vi "信号光谱2_test.vi"() -> ()   [LabVIEW 2018]
uses:
  <vilib>/Analysis/NI_AALBase.lvlib
  <vilib>/Utility/file.llb/Write Delimited Spreadsheet (DBL).vi
panel:
  in  "端口":u16
  in  "地址":string
  out "configure error out":errorcluster
  out "最终存储路径":path
  in  "停止程序":bool
  in  "上升下降沿/s":dbl format="%.2p"
  in  "延时/s":dbl format="%.2p"
  in  "占空比/%":dbl=3.0 format="%.2p"
  in  "高电平/V":dbl=4.0 format="%.2p"
  in  "频率/Hz":dbl=100.0 format="%.3p"
  in  "低电平/V":dbl min=0.0 max=5.0 format="%.2p"
  in  "设置参数":bool
  out "output control error  4":errorcluster
  in  "低电平持续输出":bool
  in  "Output 1":bool
  out "output control error  5":errorcluster
  in  "脉冲作用时间/s":dbl=1.0
  in  "测量高电平/V":dbl=4.0
  out "output control error  2":errorcluster
  in  "测量次数":i32=1
  in  "开始测量":bool
  in  "上升下降沿":i32(ring)=1 items=["上升沿", "下降沿"]
  in  "channel输出口":i32(ring) items=["Channel 1", "Channel 2"]
  in  "输出信号波形":u16(ring) items=["Pulse"]
  out "output control error  3":errorcluster
  out "Output":bool
  in  "VISA 信号发生器":refnum<visa-resource-name>="USB0::0x1AB1::0x0641::DG4E192200870::INSTR"
  out "Spectrum":cluster{"Y":dbl[], "Y":dbl[]}[](graph)
  in  "计数器":dbl=720.0
  out "波长范围":dbl[](array[numeric])
  in  "选项卡控件":enum32{"IHR 550", "CCD"}(tab)
  in  "Move To\nTarget Positions":bool
  out "Current UniqueID":string="Mono4"
  in  "Mono ID":string(combo)="Mono1"
  in  "Connect":bool
  out "Initialized JY":bool=TRUE
  in  "Force\nInitialization":bool
  in  "Target Grating":string(combo)="2"
  out "Current Description":string="1" caption="Description"
  out "Grating Index":i32=1
  out "Current Grating":dbl=1200.0
  out "Units":string="nm"
  out "Current WL":dbl=897.9988
  out "Exit Mirror\nPosition":i32(ring)=2 items=["EntranceMirror", "ExitMirror", "Front", "Side"]
  out "Entrance Mirror\nPosition":i32(ring)=2 items=["EntranceMirror", "ExitMirror", "Front", "Side"]
  out "Units 2":string="mm"
  out "Front Entrance":dbl
  in  "Target WL":dbl=2670.0
  in  "Exit Mirror":u16(ring)=3 caption="Target Position Exit Mirror" items=["Front"=2, "Side"=3]
  in  "Entrance Mirror":u16(ring)=2 caption="Target Position\nEntrance Mirror" items=["Front"=2, "Side"=3]
  in  "Target\nFront Entrance":dbl=1.0
  in  "Commande tab":T1(tab)
  in  "Area Number to Display":i32
  in  "Reformat":bool
  in  "GAIN":u16(ring)=2 caption="Device Name" items=["High Light", "Best Dynamic Range", "High Sensitivity"]
  in  "ADC":u16(ring) caption="Device Name" items=["20 kHz       ", " 1 MHz       ", " 1 MHz Ultra "]
  in  "Number of Areas :":u16=1 min=1 step=1
  in  "Integration time (ms) :":i32=5000
  out "Uniques ID":u16(ring) items=["CCD1", "CCD2"]
  in  "Device Name":u16(ring) items=["Synapse CCD (Lateral)", "Synapse_IGA (Axial)"]
  in  "Signal type :":enum16{"TTL Rising Edge", "TTL Falling Edge"}(ring)=enum."TTL Falling Edge"
  in  "Trigger Type :":u16(ring) items=["On Start"=1, "Per Acquisition"=2]
  in  "trigSigTypeString":string
  in  "trigEventString":string
  in  "Enable InputTriggers :":bool
  in  "Number of Cleans":i32=1
  in  "MultiAcqShutterMode":i32(ring)=3 items=["Open For All Spectra"=1, "Open for Each Spectrum"=3]
  in  "Accumulations:":u16=10 min=1 step=1
  in  "Multi Accumulation mode:":bool
  out "Y Pixels:":i32=256
  out "DataSize":i32=1024
  out "X Pixels:":i32=1024
  out "Firmware\nVersion":string="V1.20 CCD_4000"
  out "initialized ?":bool=TRUE
  in  "Continuous":bool
  in  "CCD Busy":bool
  out "indicator":string="Ready !"
  in  "initialize":bool
  in  "ShutterOpen":bool=TRUE caption="Shutter enable"
  in  "Save Backlight":bool
  in  "Acquire":bool
  in  "Temperature":bool
  in  "Setup":bool
  in  "起始波长":dbl=2406.79
  in  "终止波长":dbl=2919.91
  out "Acq Time(ms)":u32=3401
  in  "Close":bool=TRUE
  out "JYCCDLib.IJYCCDReqd":refnum<k7>
  out "areas :":i32[][](array[numeric])=[[1], [1], [1], [1024], [256], [1], [256]]
  in  "Constante de condition\n(Voir l'aide contextuelle)":bool
  out "temp graph":dbl(graph)=-134.538067
  out "ADC Number":i32[](array[numeric])=[0, 1, 2, 3, 4]
  out "Gain Number":i32[](array[numeric])=[10, 11, 12, 13, 8, 2]
  out "trigAddress":i32
  out "Data":i32[][](graph)
  out "error out":errorcluster
  out "Gratings":dbl[](array[numeric])=[1200.0, 300.0]
  out "Backlight":i32[][](graph)
  out "data 2":i32[][](graph)
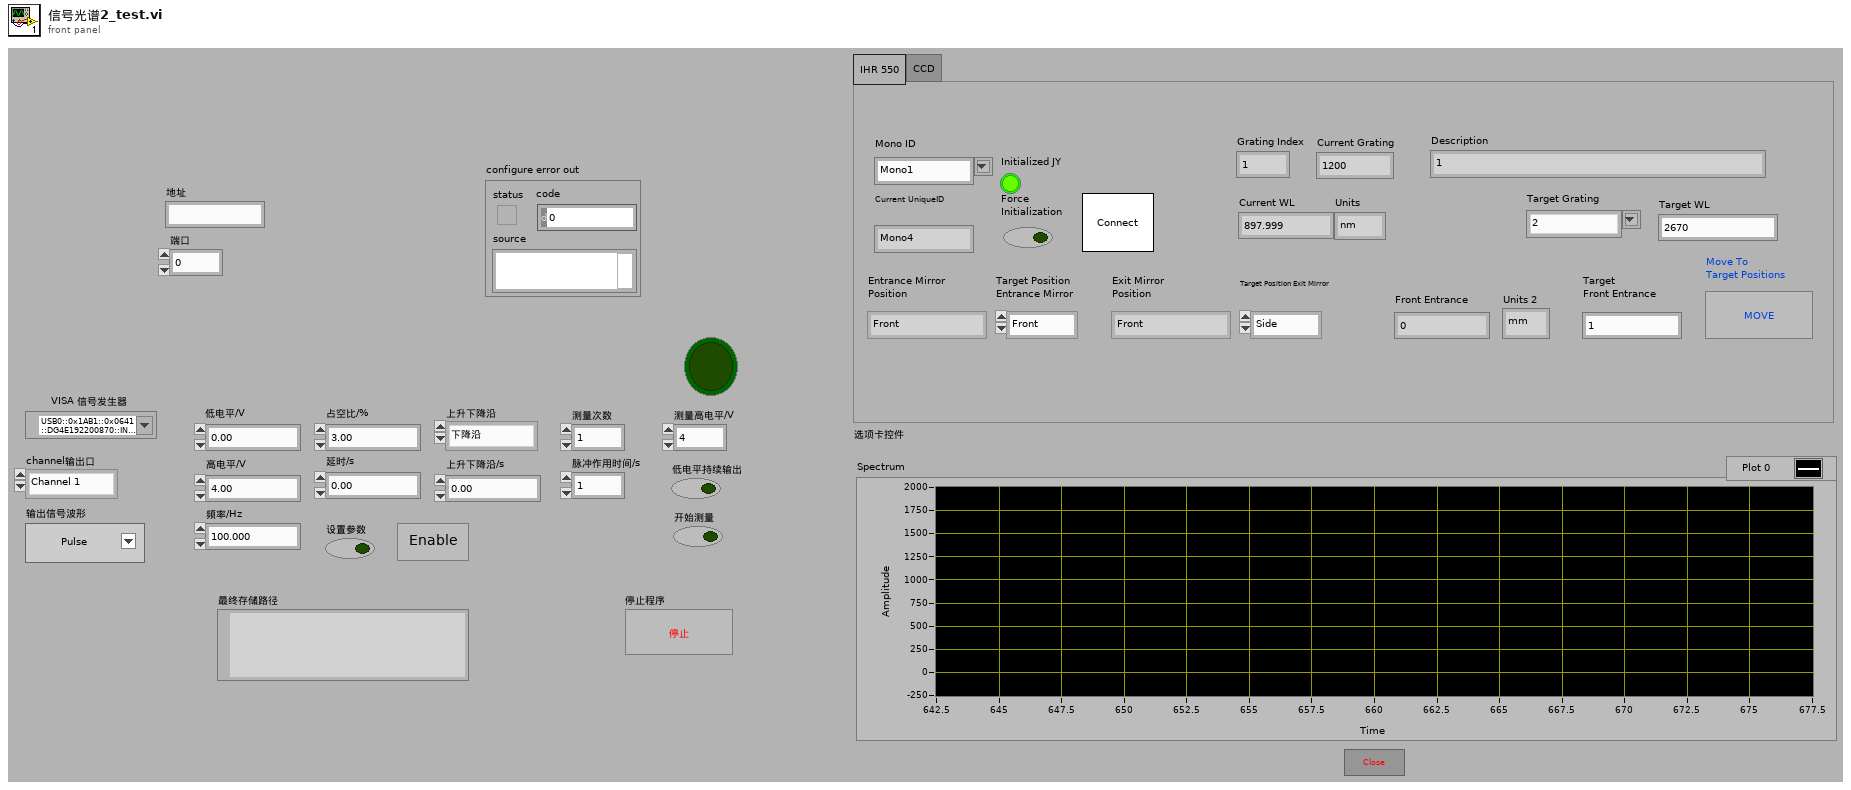
[diagram p1: front panel]
types:
  T1 = enum32{"Settings", "Trigger In", "Multi-Accu.", "Infos"}
  T2 = enum8{"Enabled", "Disabled", "Disabled and Grayed Out"}
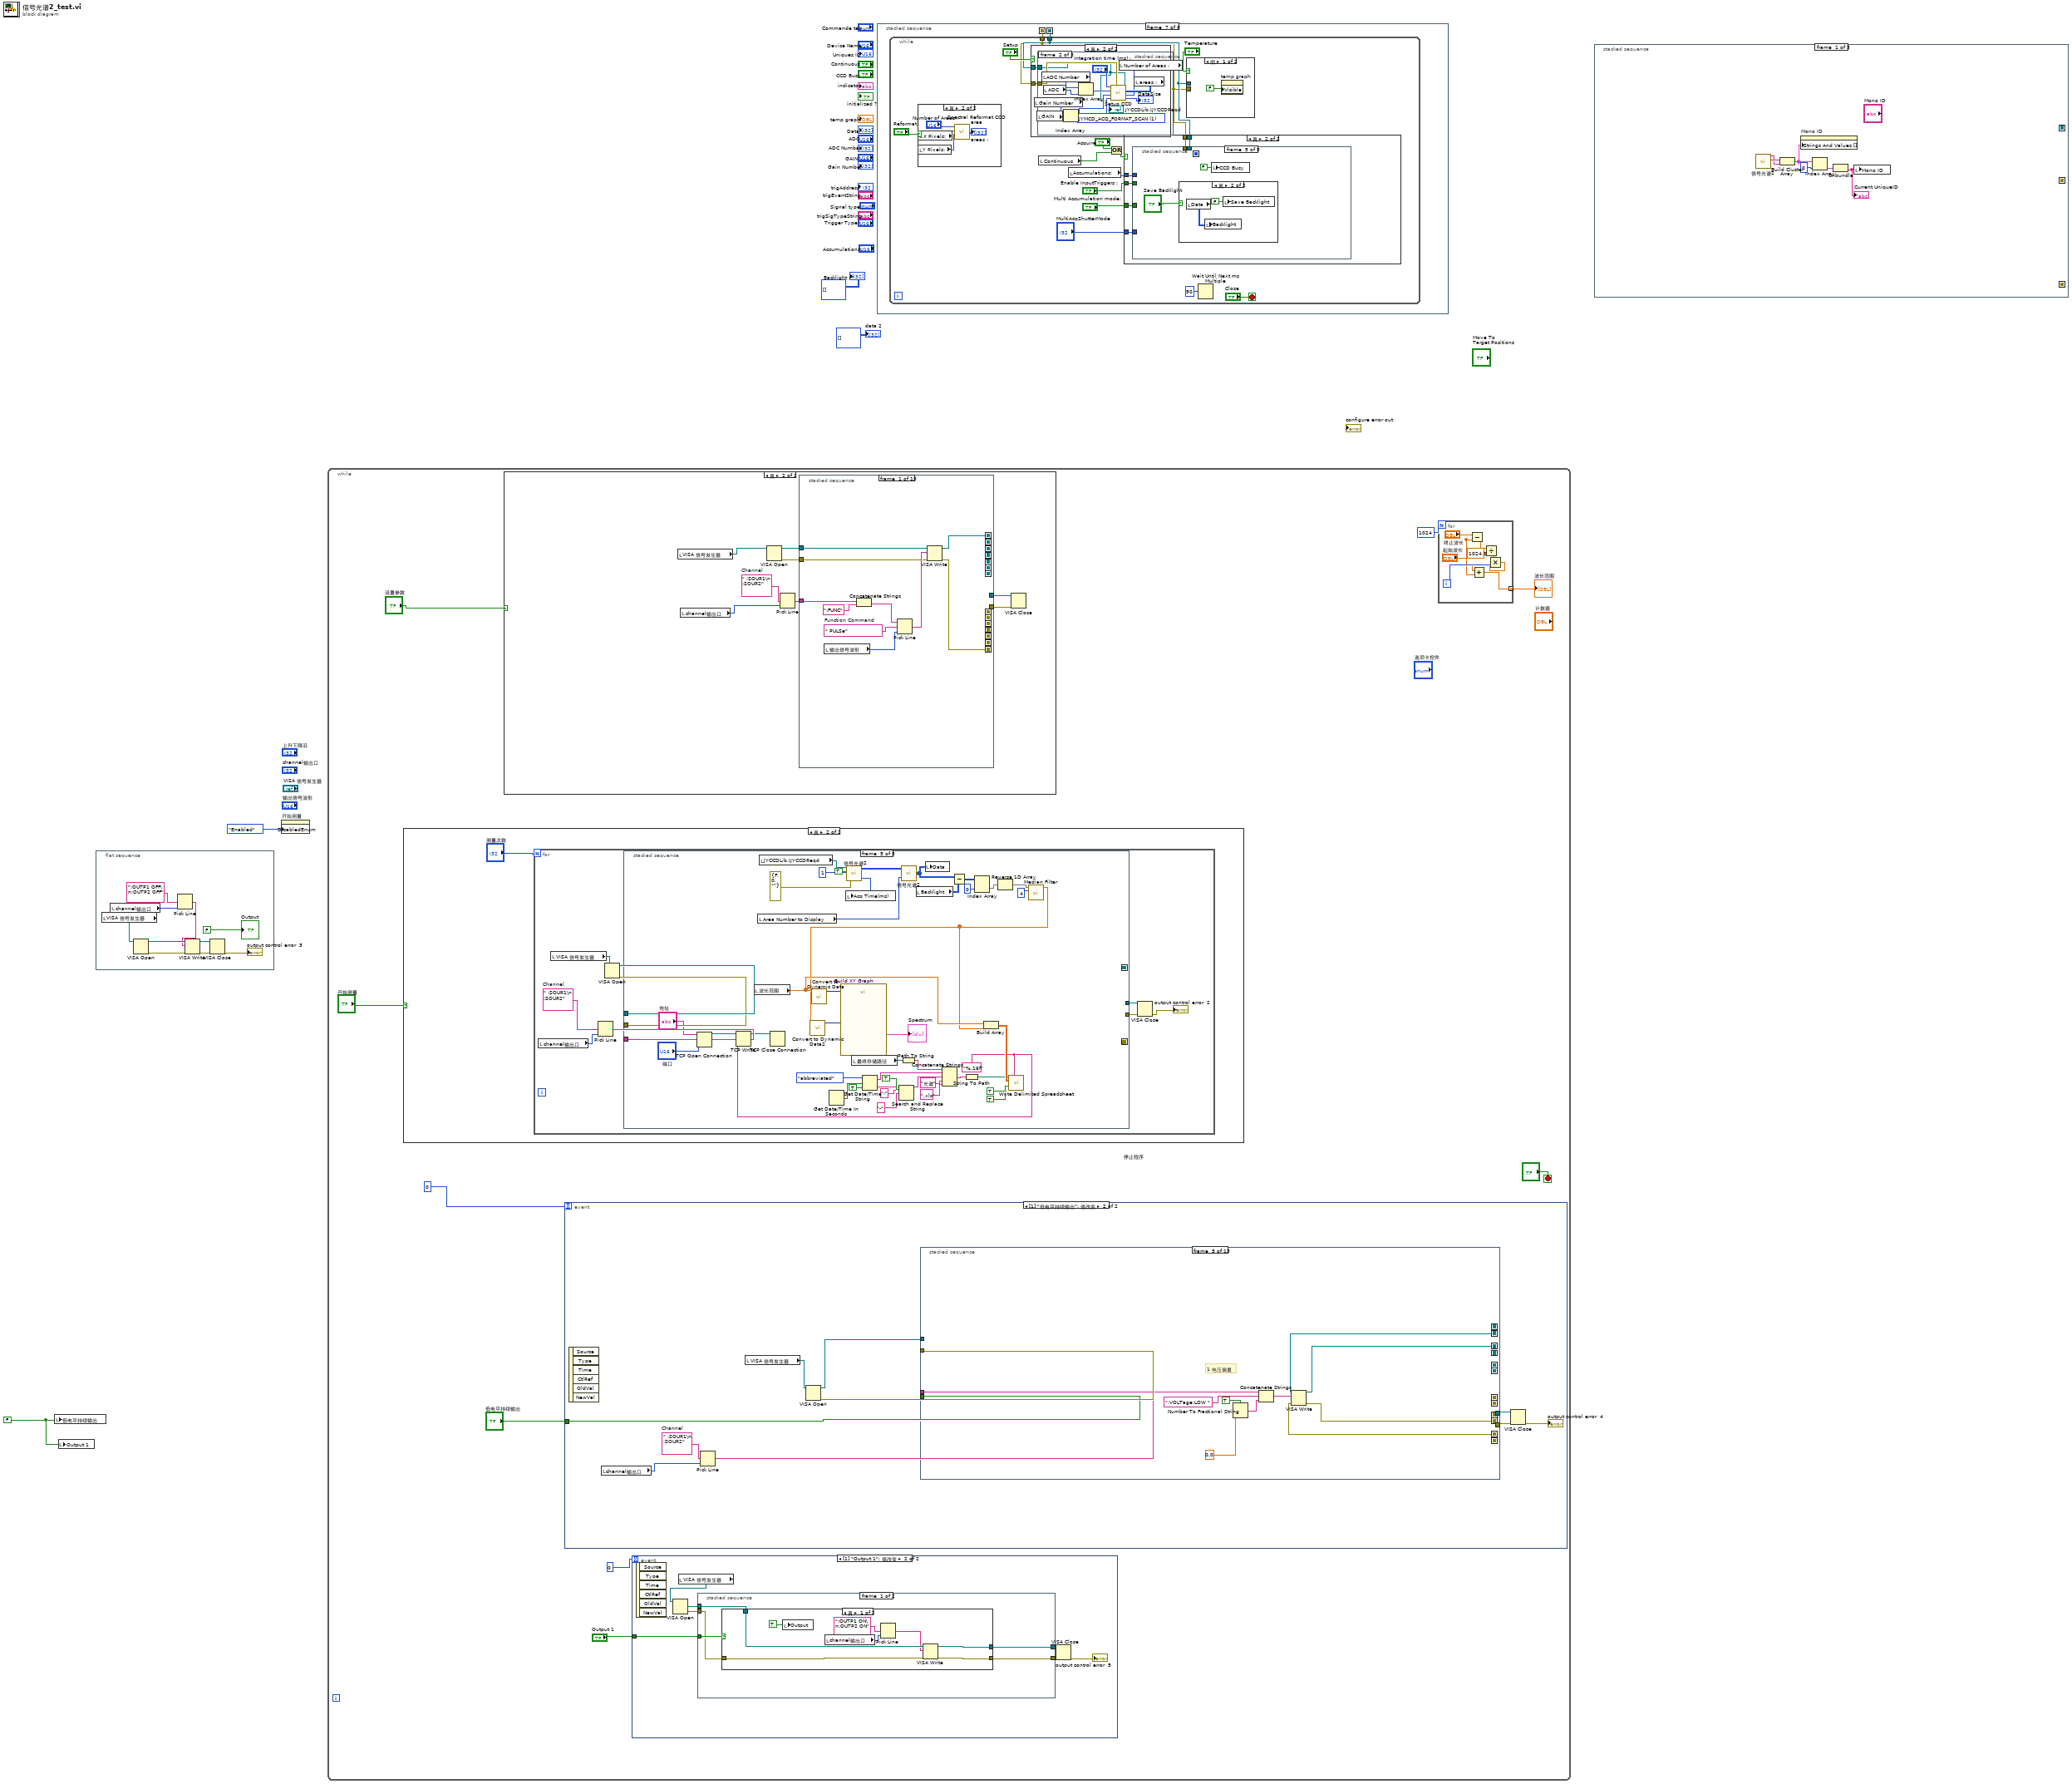
[diagram p0: block diagram]
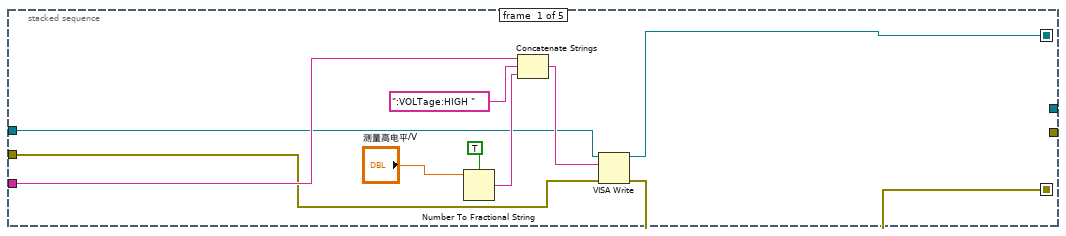
[diagram p3: hidden frame]
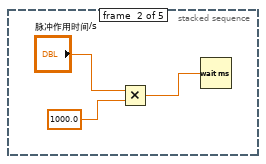
[diagram p4: hidden frame]
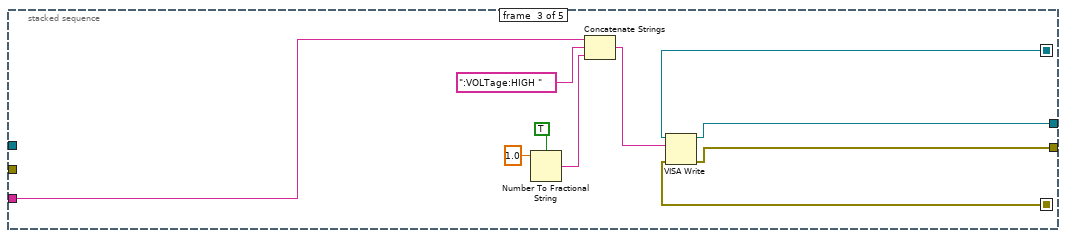
[diagram p5: hidden frame]
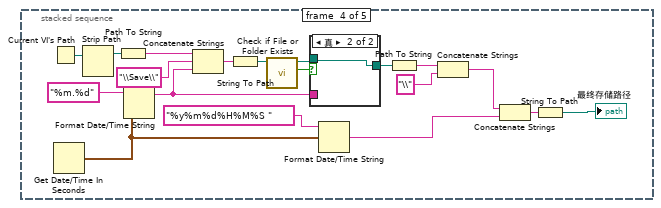
[diagram p6: hidden frame]
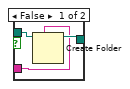
[diagram p7: hidden frame]
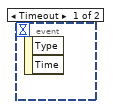
[diagram p8: hidden frame]
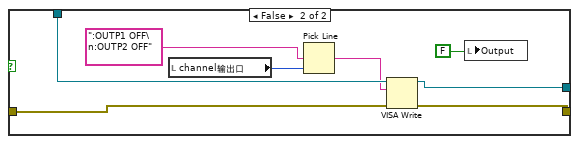
[diagram p9: hidden frame]
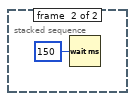
[diagram p10: hidden frame]
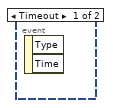
[diagram p11: hidden frame]
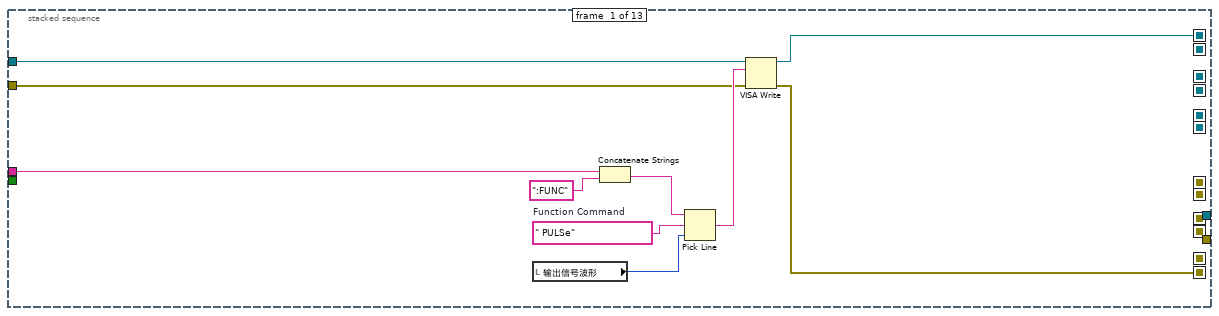
[diagram p12: hidden frame]
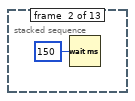
[diagram p13: hidden frame]
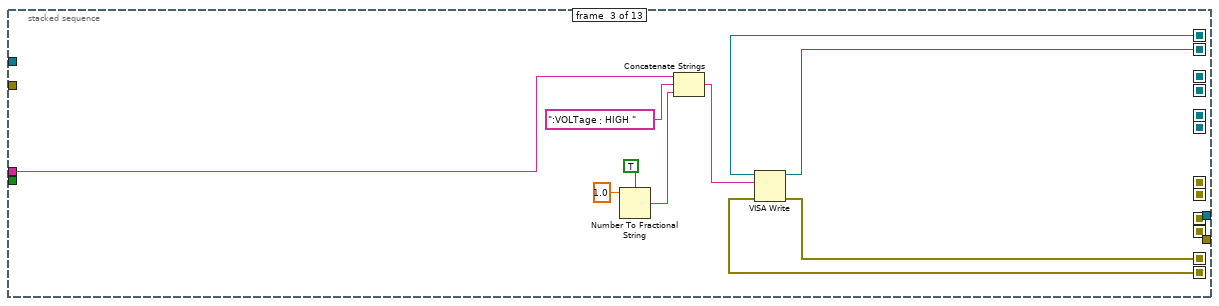
[diagram p14: hidden frame]
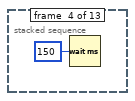
[diagram p15: hidden frame]
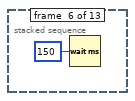
[diagram p16: hidden frame]
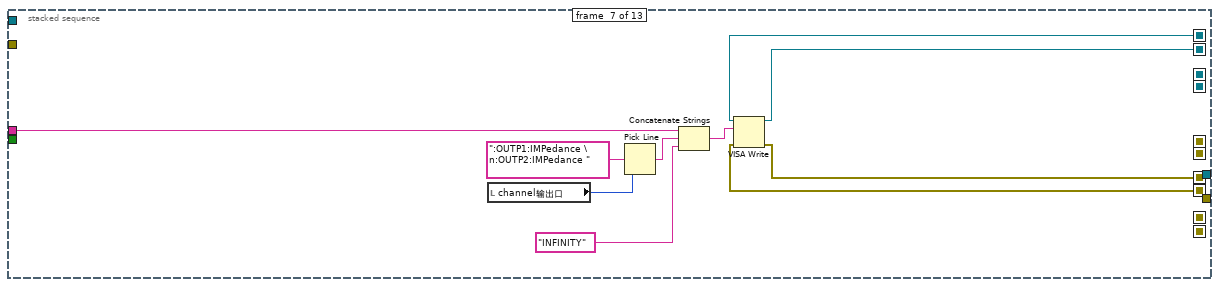
[diagram p17: hidden frame]
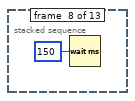
[diagram p18: hidden frame]
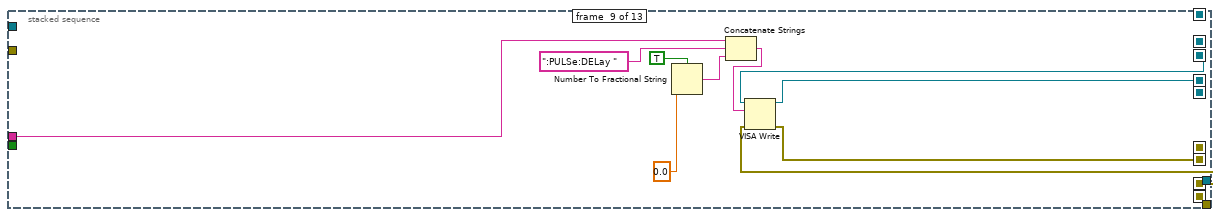
[diagram p19: hidden frame]
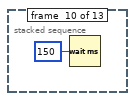
[diagram p20: hidden frame]
diagram:
  w1 = FALSE
  n1 = local write "低电平持续输出"(w1) -> ()
  n2 = local write "Output 1"(w1) -> ()
  n3 = flat-sequence {
    frame #0 {
      n4 = local read "VISA 信号发生器"() -> (w8:refnum<visa-resource-name>)
      n5 = local read "channel输出口"() -> (w6:i32)
      n6 = VISA Open(VISA resource name=w8) -> (VISA resource name=w14:refnum<visa-resource-name>, error out=w13:errorcluster)  [unwired: 4 in]
      n7 = Pick Line(multi-line string=":OUTP1 OFF\n:OUTP2 OFF" ("write buffer"), line index=w6) -> (output string=w5:string)  [unwired: 1 in]
      n8 = VISA Write(VISA resource name=w14, write buffer=w5, error in (no error)=w13) -> (VISA resource name out=w11:refnum<visa-resource-name>, error out=w10:errorcluster)  [unwired: 1 out]
      n9 = VISA Close(VISA resource name=w11, error in (no error)=w10) -> (error out=→"output control error  3":errorcluster)
      "Output" <- FALSE ("布尔")
    }
  }
  n10 = property on="开始测量" class="Bool"("DisabledEnum"=T2."Enabled" ("禁用")) -> ()  [unwired: 2 in, 2 out]
  n11 = while {
    stop <- "停止程序" stop-if-true
    n12 = case shown="真" "开始测量" {
      frame False {
      }
      frame True {
        n13 = for {
          N: "测量次数" -> [_]
          w34 = " :SOUR1\n :SOUR2"  # Channel
          n14 = local read "channel输出口"() -> (w35:i32)
          n15 = local read "VISA 信号发生器"() -> (w41:refnum<visa-resource-name>)
          n16 = Pick Line(multi-line string=w34, line index=w35) -> (output string=w33:string)  [unwired: 1 in]
          n17 = VISA Open(VISA resource name=w41) -> (VISA resource name=w40:refnum<visa-resource-name>, error out=w39:errorcluster)  [unwired: 4 in]
          n18 = stacked-sequence {
            seq-local: [w44 _ _ _ _] -> [_ _ w57 _ _]
            seq-local: [w43 _ _ _ _] -> [_ _ w56 _ _]
            tunnel: w40 -> [w46 _ _ _ _]
            tunnel: w39 -> [w45 _ _ _ _]
            tunnel: [_ _ w59 _ _] -> w38
            tunnel: [_ _ w58 _ _] -> w37
            tunnel: w33 -> [w47 _ w55 _ _]
            frame #0 {
              n19 = Number To Fractional String(use system decimal point (T)=TRUE ("使用系统小数点(T)"), number="测量高电平/V") -> (F-format string=w49:string)  [unwired: 2 in]
              n20 = Concatenate Strings ("连接字符串")(w47, ":VOLTage:HIGH ", w49) -> (w48:string)
              n21 = VISA Write(VISA resource name=w46, write buffer=w48, error in (no error)=w45) -> (VISA resource name out=w44:refnum<visa-resource-name>, error out=w43:errorcluster)  [unwired: 1 out]
            }
            frame #1 {
              n22 = Multiply(x="脉冲作用时间/s", y=1000.0) -> (x*y=w52:dbl)
              n23 = Wait (ms)(milliseconds to wait=w52) -> ()  [unwired: 1 out]
            }
            frame #2 {
              n24 = Number To Fractional String(use system decimal point (T)=TRUE ("使用系统小数点(T)"), number=1.0 ("数字")) -> (F-format string=w62:string)  [unwired: 2 in]
              n25 = Concatenate Strings ("连接字符串")(w55, ":VOLTage:HIGH ", w62) -> (w61:string)
              n26 = VISA Write(VISA resource name=w57, write buffer=w61, error in (no error)=w56) -> (VISA resource name out=w59:refnum<visa-resource-name>, error out=w58:errorcluster)  [unwired: 1 out]
            }
            frame #3 {
              n27 = Current VI's Path() -> (path=w70:path)
              n28 = Get Date/Time In Seconds() -> (seconds since 1Jan1904=w72:timestamp)
              n29 = Strip Path(path=w70) -> (stripped path=w71:path)  [unwired: 1 out]
              n30 = Path To String(path=w71) -> (string=w73:string)
              n31 = Format Date/Time String(time format string (%c)="%m.%d" ("时间格式字符串(%c)"), seconds (now)=w72) -> (date/time string=w79:string)  [unwired: 1 in]
              n32 = Concatenate Strings(w73, "\\Save\\" ("字符串"), w79) -> (w74:string)
              n33 = String To Path(string=w74) -> (path=w75:path)
              n34 = call <vilib>:"Check if File or Folder Exists.vi"("path"=w75) -> ("file or folder exists?"=w76:bool, "dup path"=w78:path)  [unwired: 8 in, 1 out]
              n35 = case shown="真" w76 {
                tunnel: [w86 w87] -> w77
                tunnel: w78 -> [w85 w87]
                tunnel: w79 -> [w84 _]
                frame False {
                  n36 = Create Folder(prompt (Create Folder)=w84, path (use dialog)=w85) -> (created path=w86:path)  [unwired: 1 in, 2 out]
                }
                frame True {
                }
              }
              n37 = Format Date/Time String(time format string (%c)="%y%m%d%H%M%S " ("时间格式字符串(%c)"), seconds (now)=w72) -> (date/time string=w82:string)  [unwired: 1 in]
              n38 = Path To String(path=w77) -> (string=w80:string)
              n39 = Concatenate Strings(w80, "\\" ("字符串")) -> (w81:string)
              n40 = Concatenate Strings(w81, w82) -> (w69:string)
              n41 = String To Path(string=w69) -> (path=→"最终存储路径":path)
            }
            frame #4 {
              w90 = "%.16f" ("format (%.3f)")
              n42 = TCP Open Connection(address="地址", remote port or service name="端口") -> (connection ID=w93:refnum<k5>)  [unwired: 3 in, 1 out]
              n43 = TCP Write(connection ID=w93, data in=w90) -> (connection ID out=w92:refnum<k5>)  [unwired: 2 in, 2 out]
              n44 = local read "波长范围"() -> (w129:dbl[])
              n45 = local read "Area Number to Display"() -> (w98:i32)
              n46 = local read "JYCCDLib.IJYCCDReqd"() -> (w94:refnum<k7>)
              n47 = TCP Close Connection(connection ID=w92) -> ()  [unwired: 2 in, 2 out]
              n48 = call "Convert to Dynamic Data"("Array"=w129) -> ("Dynamic Data Type"=w107:dynamicdata)  [unwired: 3 in]
              n49 = Get Date/Time In Seconds() -> (seconds since 1Jan1904=w112:timestamp)
              n50 = call "信号光谱2.vi"("error in"=errorcluster {"status"=FALSE, "code"=0, "source"=""}, "Accumulations:"=u16 1, "ShutterOpen"=TRUE, "JYCCDLib.IJYCCDReqd"=w94) -> ("Acq Time(ms)"=w100:u32, "Array Out"=w99:i32[][][])  [unwired: 1 out]
              n51 = local write "Acq Time(ms)"(w100) -> ()
              n52 = local read "最终存储路径"() -> (w124:path)
              n53 = Get Date/Time String(date format (0)=enum16{"short", "long", "abbreviated"}."abbreviated" ("日期格式(0)"), seconds (now)=w112, want seconds? (F)=TRUE ("需要秒？(F)")) -> (date string=w120:string, time string=w115:string)
              n54 = Search and Replace String(replace all?=TRUE ("替换全部？(F)"), input string=w115, search string=":" ("搜索字符串"), replace string="-" ("替换字符串(\"\")")) -> (result string=w119:string)  [unwired: 4 in, 3 out]
              n55 = call "信号光谱2.vi"("Area Number"=w98, "Array In"=w99) -> ("Array Out"=w101:i32[][])
              n56 = Path To String(path=w124) -> (string=w109:string)
              n57 = local read "Backlight"() -> (w102:i32[][])
              n58 = local write "Data"(w101) -> ()
              n59 = Concatenate Strings(w109, w120, w119, "光谱" ("字符串"), ".xls" ("字符串")) -> (w91:string)
              n60 = Subtract(x=w101, y=w102) -> (x-y=w103:i32[][])
              n61 = String To Path(string=w91) -> (path=w123:path)
              n62 = Index Array(array=w103, index (row)=0 ("索引 (行)")) -> (element=w125:i32[])  [unwired: 1 in]
              n63 = Reverse 1D Array(array=w125) -> (reversed array=w126:i32[])
              n64 = call <vilib>:"Median Filter.vi"("left rank"=4, "X"=w126) -> ("Filtered X"=w128:dbl[])  [unwired: 8 in, 1 out]
              n65 = call "Convert to Dynamic Data2"("Array"=w128) -> ("Dynamic Data Type"=w106:dynamicdata)  [unwired: 3 in]
              n66 = call "Build XY Graph"("Y Input"=w106, "X Input"=w107) -> ("XY Graph"=→"Spectrum":cluster{"Y":dbl[], "Y":dbl[]}[])  [unwired: 8 in, 1 out]
              n67 = Build Array(w129, w128) -> (w127:dbl[][])
              n68 = call-poly <vilib>:"Write Delimited Spreadsheet.vi"("file path (dialog if empty)"=w123, "format (%.3f)"=w90, "2D data"=w127, "append to file? (new file:F)"=TRUE ("append to file? (F)"), "transpose? (no:F)"=TRUE ("transpose? (F)")) -> ()  [unwired: 9 in, 2 out]
            }
          }
          n69 = VISA Close(VISA resource name=w38, error in (no error)=w37) -> (error out=→"output control error  2":errorcluster)
        }
      }
    }
    n70 = case shown="真" "设置参数" {
      frame False {
      }
      frame True {
        w264 = " :SOUR1\n :SOUR2"  # Channel
        n71 = local read "VISA 信号发生器"() -> (w260:refnum<visa-resource-name>)
        n72 = local read "channel输出口"() -> (w259:i32)
        n73 = VISA Open(VISA resource name=w260) -> (VISA resource name=w266:refnum<visa-resource-name>, error out=w267:errorcluster)  [unwired: 4 in]
        n74 = Pick Line(multi-line string=w264, line index=w259) -> (output string=w263:string)  [unwired: 1 in]
        n75 = stacked-sequence {
          seq-local: [w272 _ _ _ _ _ _ _ _ _ _ _ _ _ _] -> [_ _ w287 _ _ _ _ _ _ _ _ _ _ _ _]
          seq-local: [w271 _ _ _ _ _ _ _ _ _ _ _ _ _ _] -> [_ _ w286 _ _ _ _ _ _ _ w325 _ _ _ _]
          seq-local: [_ _ w285 _ _ _ _ _ _ _ _ _ _ _ _] -> [_ _ _ _ w296 _ _ _ _ _ _ _ _ _ _]
          seq-local: [_ _ w284 _ _ _ _ _ _ _ _ _ _ _ _] -> [_ _ _ _ w295 _ _ _ _ _ _ _ _ _ _]
          seq-local: [_ _ _ _ w294 _ _ _ _ _ _ _ _ _ _] -> [_ _ _ _ _ _ w302 _ _ _ _ _ _ _ _]
          seq-local: [_ _ _ _ w291 _ _ _ _ _ _ _ _ _ _] -> [_ _ _ _ _ _ w301 _ _ _ _ _ _ _ _]
          seq-local: [_ _ _ _ _ _ w309 _ _ _ _ _ _ _ _] -> [_ _ _ _ _ _ _ _ w320 _ _ _ _ _ _]
          seq-local: [_ _ _ _ _ _ w308 _ _ _ _ _ _ _ _] -> [_ _ _ _ _ _ _ _ w319 _ _ _ _ _ _]
          seq-local: [_ _ _ _ _ _ _ _ w313 _ _ _ _ _ _] -> [_ _ _ _ _ _ _ _ _ _ w326 _ _ _ _]
          seq-local: [_ _ _ _ _ _ _ _ w312 _ _ _ _ _ _] -> [_ _ _ _ _ _ _ _ _ _ _ _ _ _ _]
          seq-local: [_ _ _ _ _ _ _ _ _ _ w322 _ _ _ _] -> [_ _ _ _ _ _ _ _ _ _ _ _ w336 _ _]
          seq-local: [_ _ _ _ _ _ _ _ _ _ w323 _ _ _ _] -> [_ _ _ _ _ _ _ _ _ _ _ _ w335 _ _]
          seq-local: [_ _ _ _ _ _ _ _ _ _ _ _ w334 _ _] -> [_ _ _ _ _ _ _ _ _ _ _ _ _ _ w347]
          seq-local: [_ _ _ _ _ _ _ _ _ _ _ _ w333 _ _] -> [_ _ _ _ _ _ _ _ _ _ _ _ _ _ w346]
          tunnel: w266 -> [w277 _ _ _ _ _ _ _ _ _ _ _ _ _ _]
          tunnel: w267 -> [w270 _ _ _ _ _ _ _ _ _ _ _ _ _ _]
          tunnel: w263 -> [w269 _ w283 _ w290 _ w306 _ w317 _ w327 _ w337 _ w350]
          tunnel: [_ _ _ _ _ _ _ _ _ _ _ _ _ _ w345] -> w262
          tunnel: [_ _ _ _ _ _ _ _ _ _ _ _ _ _ w344] -> w261
          frame #0 {
            w274 = " PULSe"  # Function Command
            n76 = local read "输出信号波形"() -> (w268:u16)
            n77 = Concatenate Strings(w269, ":FUNC" ("string (\"\")")) -> (w275:string)
            n78 = Pick Line(string ("")=w275, multi-line string=w274, line index=w268) -> (output string=w273:string)
            n79 = VISA Write(VISA resource name=w277, write buffer=w273, error in (no error)=w270) -> (VISA resource name out=w272:refnum<visa-resource-name>, error out=w271:errorcluster)  [unwired: 1 out]
          }
          frame #1 {
            n80 = Wait (ms)(milliseconds to wait=u32 150) -> ()  [unwired: 1 out]
          }
          frame #2 {
            n81 = Number To Fractional String(use system decimal point (T)=TRUE ("使用系统小数点(T)"), number="低电平/V") -> (F-format string=w281:string)  [unwired: 2 in]
            n82 = Concatenate Strings ("连接字符串")(w283, ":VOLTage:LOW ", w281) -> (w280:string)
            n83 = VISA Write(VISA resource name=w287, write buffer=w280, error in (no error)=w286) -> (VISA resource name out=w285:refnum<visa-resource-name>, error out=w284:errorcluster)  [unwired: 1 out]
          }
          frame #3 {
            n84 = Wait (ms)(milliseconds to wait=u32 150) -> ()  [unwired: 1 out]
          }
          frame #4 {
            # "1 频率"
            n85 = Concatenate Strings(w290, ":FREQ ") -> (w297:string)
            n86 = Format Into String ("格式化写入字符串")(initial string=w297, "频率/Hz") -> (resulting string=w298:string)  [unwired: 2 in, 1 out]
            n87 = VISA Write(VISA resource name=w296, write buffer=w298, error in (no error)=w295) -> (VISA resource name out=w294:refnum<visa-resource-name>, error out=w291:errorcluster)  [unwired: 1 out]
          }
          frame #5 {
            n88 = Wait (ms)(milliseconds to wait=u32 150) -> ()  [unwired: 1 out]
          }
          frame #6 {
            n89 = Number To Fractional String(use system decimal point (T)=TRUE ("使用系统小数点(T)"), number="高电平/V") -> (F-format string=w303:string)  [unwired: 2 in]
            n90 = Concatenate Strings(w306, ":VOLTage:HIGH ", w303) -> (w305:string)
            n91 = VISA Write(VISA resource name=w302, write buffer=w305, error in (no error)=w301) -> (VISA resource name out=w309:refnum<visa-resource-name>, error out=w308:errorcluster)  [unwired: 1 out]
          }
          frame #7 {
            n92 = Wait (ms)(milliseconds to wait=u32 150) -> ()  [unwired: 1 out]
          }
          frame #8 {
            n93 = local read "channel输出口"() -> (w315:i32)
            n94 = Pick Line(multi-line string=":OUTP1:IMPedance \n:OUTP2:IMPedance " ("write buffer"), line index=w315) -> (output string=w314:string)  [unwired: 1 in]
            n95 = Concatenate Strings ("连接字符串")(w317, w314, "INFINITY") -> (w318:string)
            n96 = VISA Write(VISA resource name=w320, write buffer=w318, error in (no error)=w319) -> (VISA resource name out=w313:refnum<visa-resource-name>, error out=w312:errorcluster)  [unwired: 1 out]
          }
          frame #9 {
            n97 = Wait (ms)(milliseconds to wait=u32 150) -> ()  [unwired: 1 out]
          }
          frame #10 {
            n98 = Number To Fractional String(use system decimal point (T)=TRUE ("使用系统小数点(T)"), number="占空比/%") -> (F-format string=w329:string)  [unwired: 2 in]
            n99 = Concatenate Strings(w327, ":PULSe:DCYCle ", w329) -> (w324:string)
            n100 = VISA Write(VISA resource name=w326, write buffer=w324, error in (no error)=w325) -> (VISA resource name out=w322:refnum<visa-resource-name>, error out=w323:errorcluster)  [unwired: 1 out]
          }
          frame #11 {
            n101 = Wait (ms)(milliseconds to wait=u32 150) -> ()  [unwired: 1 out]
          }
          frame #12 {
            n102 = Number To Fractional String(use system decimal point (T)=TRUE ("使用系统小数点(T)"), number="延时/s") -> (F-format string=w340:string)  [unwired: 2 in]
            n103 = Concatenate Strings(w337, ":PULSe:DELay ", w340) -> (w338:string)
            n104 = VISA Write(VISA resource name=w336, write buffer=w338, error in (no error)=w335) -> (VISA resource name out=w334:refnum<visa-resource-name>, error out=w333:errorcluster)  [unwired: 1 out]
          }
          frame #13 {
            n105 = Wait (ms)(milliseconds to wait=u32 150) -> ()  [unwired: 1 out]
          }
          frame #14 {
            w351 = ":LEADing\n:TRAiling "  # Channel
            w356 = ":PULSe:TRANsition"  # VOLTage:Offset
            n106 = local read "上升下降沿"() -> (w352:i32)
            n107 = Pick Line(multi-line string=w351, line index=w352) -> (output string=w348:string)  [unwired: 1 in]
            n108 = Number To Fractional String(use system decimal point (T)=TRUE ("使用系统小数点(T)"), number="上升下降沿/s") -> (F-format string=w349:string)  [unwired: 2 in]
            n109 = Concatenate Strings(w350, w356, w348, w349) -> (w353:string)
            n110 = VISA Write(VISA resource name=w347, write buffer=w353, error in (no error)=w346) -> (VISA resource name out=w345:refnum<visa-resource-name>, error out=w344:errorcluster)  [unwired: 1 out]
          }
        }
        n111 = VISA Close(VISA resource name=w262, error in (no error)=w261) -> (error out=w265:errorcluster)
      }
    }
    n112 = event shown="[1] \"低电平持续输出\": 值改变" {
      selector: _ -> [_ _]
      dyn-events: _ -> [_ _]
      timeout: u32 0 ("Time") -> [_ _]
      tunnel: "低电平持续输出" -> [_ w159]
      event Timeout {
        n113 = event-data() -> ()  [unwired: 1 in, 2 out]
      }
      event "低电平持续输出": Value Change {
        w163 = " :SOUR1\n :SOUR2"  # Channel
        n114 = event-data() -> ()  [unwired: 1 in, 6 out]
        n115 = local read "channel输出口"() -> (w164:i32)
        n116 = Pick Line(multi-line string=w163, line index=w164) -> (output string=w162:string)  [unwired: 1 in]
        n117 = local read "VISA 信号发生器"() -> (w167:refnum<visa-resource-name>)
        n118 = VISA Open(VISA resource name=w167) -> (VISA resource name=w166:refnum<visa-resource-name>, error out=w165:errorcluster)  [unwired: 4 in]
        n119 = stacked-sequence {
          seq-local: [w173 _ _ _ _ _ _ _ _ _ _ _ _] -> [_ _ w188 _ _ _ _ _ _ _ _ _ _]
          seq-local: [w172 _ _ _ _ _ _ _ _ _ _ _ _] -> [_ _ w187 _ _ _ _ _ _ _ _ _ _]
          seq-local: [_ _ w186 _ _ _ _ _ _ _ _ _ _] -> [_ _ _ _ w191 _ _ _ _ _ _ _ _]
          seq-local: [_ _ w185 _ _ _ _ _ _ _ _ _ _] -> [_ _ _ _ w192 _ _ _ _ _ _ _ _]
          seq-local: [_ _ _ _ w200 _ _ _ _ _ _ _ _] -> [_ _ _ _ _ _ w211 _ _ _ _ _ _]
          seq-local: [_ _ _ _ w199 _ _ _ _ _ _ _ _] -> [_ _ _ _ _ _ w210 _ _ _ _ _ _]
          seq-local: [_ _ _ _ _ _ w204 _ _ _ _ _ _] -> [_ _ _ _ _ _ _ _ w214 _ _ _ _]
          seq-local: [_ _ _ _ _ _ w203 _ _ _ _ _ _] -> [_ _ _ _ _ _ _ _ w213 _ _ _ _]
          seq-local: [_ _ _ _ _ _ _ _ w217 _ _ _ _] -> [_ _ _ _ _ _ _ _ _ _ w228 _ _]
          seq-local: [_ _ _ _ _ _ _ _ w216 _ _ _ _] -> [_ _ _ _ _ _ _ _ _ _ w227 _ _]
          seq-local: [_ _ _ _ _ _ _ _ _ _ w225 _ _] -> [_ _ _ _ _ _ _ _ _ _ _ _ w242]
          seq-local: [_ _ _ _ _ _ _ _ _ _ w224 _ _] -> [_ _ _ _ _ _ _ _ _ _ _ _ w241]
          tunnel: w166 -> [w178 _ _ _ _ _ _ _ _ _ _ _ _]
          tunnel: w165 -> [w171 _ _ _ _ _ _ _ _ _ _ _ _]
          tunnel: w162 -> [w170 _ w184 _ w197 _ w208 _ w218 _ w231 _ _]
          tunnel: [_ _ _ _ _ _ _ _ _ _ _ _ w240] -> w161
          tunnel: [_ _ _ _ _ _ _ _ _ _ _ _ w238] -> w160
          tunnel: w159 -> [_ _ _ _ _ _ _ _ _ _ _ _ w239]
          frame #0 {
            w175 = " PULSe"  # Function Command
            n120 = local read "输出信号波形"() -> (w169:u16)
            n121 = Concatenate Strings(w170, ":FUNC" ("string (\"\")")) -> (w176:string)
            n122 = Pick Line(string ("")=w176, multi-line string=w175, line index=w169) -> (output string=w174:string)
            n123 = VISA Write(VISA resource name=w178, write buffer=w174, error in (no error)=w171) -> (VISA resource name out=w173:refnum<visa-resource-name>, error out=w172:errorcluster)  [unwired: 1 out]
          }
          frame #1 {
            n124 = Wait (ms)(milliseconds to wait=u32 150) -> ()  [unwired: 1 out]
          }
          frame #2 {
            n125 = Number To Fractional String(use system decimal point (T)=TRUE ("使用系统小数点(T)"), number=1.0 ("数字")) -> (F-format string=w182:string)  [unwired: 2 in]
            n126 = Concatenate Strings ("连接字符串")(w184, ":VOLTage：HIGH ", w182) -> (w181:string)
            n127 = VISA Write(VISA resource name=w188, write buffer=w181, error in (no error)=w187) -> (VISA resource name out=w186:refnum<visa-resource-name>, error out=w185:errorcluster)  [unwired: 1 out]
          }
          frame #3 {
            n128 = Wait (ms)(milliseconds to wait=u32 150) -> ()  [unwired: 1 out]
          }
          frame #4 {
            # "1 电压偏置"
            n129 = Number To Fractional String(use system decimal point (T)=TRUE ("使用系统小数点(T)"), number=0.0 ("数字")) -> (F-format string=w195:string)  [unwired: 2 in]
            n130 = Concatenate Strings(w197, ":VOLTage:LOW ", w195) -> (w196:string)
            n131 = VISA Write(VISA resource name=w191, write buffer=w196, error in (no error)=w192) -> (VISA resource name out=w200:refnum<visa-resource-name>, error out=w199:errorcluster)  [unwired: 1 out]
          }
          frame #5 {
            n132 = Wait (ms)(milliseconds to wait=u32 150) -> ()  [unwired: 1 out]
          }
          frame #6 {
            n133 = local read "channel输出口"() -> (w206:i32)
            n134 = Pick Line(multi-line string=":OUTP1:IMPedance \n:OUTP2:IMPedance " ("write buffer"), line index=w206) -> (output string=w205:string)  [unwired: 1 in]
            n135 = Concatenate Strings ("连接字符串")(w208, w205, "INFINITY") -> (w209:string)
            n136 = VISA Write(VISA resource name=w211, write buffer=w209, error in (no error)=w210) -> (VISA resource name out=w204:refnum<visa-resource-name>, error out=w203:errorcluster)  [unwired: 1 out]
          }
          frame #7 {
            n137 = Wait (ms)(milliseconds to wait=u32 150) -> ()  [unwired: 1 out]
          }
          frame #8 {
            n138 = Number To Fractional String(use system decimal point (T)=TRUE ("使用系统小数点(T)"), number=0.0 ("数字")) -> (F-format string=w221:string)  [unwired: 2 in]
            n139 = Concatenate Strings(w218, ":PULSe:DELay ", w221) -> (w219:string)
            n140 = VISA Write(VISA resource name=w214, write buffer=w219, error in (no error)=w213) -> (VISA resource name out=w217:refnum<visa-resource-name>, error out=w216:errorcluster)  [unwired: 1 out]
          }
          frame #9 {
            n141 = Wait (ms)(milliseconds to wait=u32 150) -> ()  [unwired: 1 out]
          }
          frame #10 {
            w232 = ":LEADing\n:TRAiling "  # Channel
            w236 = ":PULSe:TRANsition"  # VOLTage:Offset
            n142 = local read "上升下降沿"() -> (w233:i32)
            n143 = Pick Line(multi-line string=w232, line index=w233) -> (output string=w229:string)  [unwired: 1 in]
            n144 = Number To Fractional String(use system decimal point (T)=TRUE ("使用系统小数点(T)"), number=0.0 ("数字")) -> (F-format string=w230:string)  [unwired: 2 in]
            n145 = Concatenate Strings(w231, w236, w229, w230) -> (w234:string)
            n146 = VISA Write(VISA resource name=w228, write buffer=w234, error in (no error)=w227) -> (VISA resource name out=w225:refnum<visa-resource-name>, error out=w224:errorcluster)  [unwired: 1 out]
          }
          frame #11 {
            n147 = Wait (ms)(milliseconds to wait=u32 150) -> ()  [unwired: 1 out]
          }
          frame #12 {
            n148 = case shown="假" w239 {
              tunnel: w242 -> [w250 w251]
              tunnel: [w249 w258] -> w238
              tunnel: w241 -> [w248 w256]
              tunnel: [w247 w257] -> w240
              frame True {
                n149 = local write "Output"(TRUE ("布尔")) -> ()
                n150 = local read "channel输出口"() -> (w244:i32)
                n151 = Pick Line(multi-line string=":OUTP1 ON\n:OUTP2 ON" ("write buffer"), line index=w244) -> (output string=w243:string)  [unwired: 1 in]
                n152 = VISA Write(VISA resource name=w250, write buffer=w243, error in (no error)=w248) -> (VISA resource name out=w247:refnum<visa-resource-name>, error out=w249:errorcluster)  [unwired: 1 out]
              }
              frame False {
                n153 = local read "channel输出口"() -> (w253:i32)
                n154 = Pick Line(multi-line string=":OUTP1 OFF\n:OUTP2 OFF" ("write buffer"), line index=w253) -> (output string=w252:string)  [unwired: 1 in]
                n155 = VISA Write(VISA resource name=w251, write buffer=w252, error in (no error)=w256) -> (VISA resource name out=w257:refnum<visa-resource-name>, error out=w258:errorcluster)  [unwired: 1 out]
                n156 = local write "Output"(FALSE ("布尔")) -> ()
              }
            }
          }
        }
        n157 = VISA Close(VISA resource name=w161, error in (no error)=w160) -> (error out=→"output control error  4":errorcluster)
      }
    }
    n158 = event shown="[1] \"Output 1\": 值改变" {
      selector: _ -> [_ _]
      dyn-events: _ -> [_ _]
      timeout: u32 0 ("Time") -> [_ _]
      tunnel: "Output 1" -> [_ w134]
      event Timeout {
        n159 = event-data() -> ()  [unwired: 1 in, 2 out]
      }
      event "Output 1": Value Change {
        n160 = event-data() -> ()  [unwired: 1 in, 6 out]
        n161 = local read "VISA 信号发生器"() -> (w130:refnum<visa-resource-name>)
        n162 = VISA Open(VISA resource name=w130) -> (VISA resource name=w133:refnum<visa-resource-name>, error out=w136:errorcluster)  [unwired: 4 in]
        n163 = stacked-sequence {
          tunnel: w134 -> [w141 _]
          tunnel: w136 -> [w140 _]
          tunnel: w133 -> [w139 _]
          tunnel: [w138 _] -> w132
          tunnel: [w137 _] -> w131
          frame #0 {
            n164 = case shown="真" w141 {
              tunnel: w139 -> [w149 w157]
              tunnel: [w148 w156] -> w137
              tunnel: w140 -> [w147 w154]
              tunnel: [w146 w155] -> w138
              frame True {
                n165 = local write "Output"(TRUE ("布尔")) -> ()
                n166 = local read "channel输出口"() -> (w143:i32)
                n167 = Pick Line(multi-line string=":OUTP1 ON\n:OUTP2 ON" ("write buffer"), line index=w143) -> (output string=w142:string)  [unwired: 1 in]
                n168 = VISA Write(VISA resource name=w149, write buffer=w142, error in (no error)=w147) -> (VISA resource name out=w146:refnum<visa-resource-name>, error out=w148:errorcluster)  [unwired: 1 out]
              }
              frame False {
                n169 = local read "channel输出口"() -> (w151:i32)
                n170 = Pick Line(multi-line string=":OUTP1 OFF\n:OUTP2 OFF" ("write buffer"), line index=w151) -> (output string=w150:string)  [unwired: 1 in]
                n171 = VISA Write(VISA resource name=w157, write buffer=w150, error in (no error)=w154) -> (VISA resource name out=w155:refnum<visa-resource-name>, error out=w156:errorcluster)  [unwired: 1 out]
                n172 = local write "Output"(FALSE ("布尔")) -> ()
              }
            }
          }
          frame #1 {
            n173 = Wait (ms)(milliseconds to wait=u32 150) -> ()  [unwired: 1 out]
          }
        }
        n174 = VISA Close(VISA resource name=w132, error in (no error)=w131) -> (error out=→"output control error  5":errorcluster)
      }
    }
    n175 = for {
      N: 1024 -> [_]
      tunnel: [w28] -> w16 mode=indexing
      i -> [w30]
      n176 = Subtract(x="终止波长", y="起始波长") -> (x-y=w26:dbl)
      n177 = Divide(x=w26, y=1024.0) -> (x/y=w24:dbl)
      n178 = Multiply(x=w24, y=w30) -> (x*y=w29:dbl)
      n179 = Add(x=w29, y="起始波长") -> (x+y=w28:dbl)
    }
    "波长范围" <- w16
  }
  n180 = stacked-sequence {
    seq-local: [_ _ _ w377 _ _ _ _] -> [_ _ _ _ w395 w415 w418 w516]
    seq-local: [_ _ _ w376 _ _ _ _] -> [_ _ _ _ w396 w416 w417 w517]
    frame #0 {
      # "initialize all variables"
      n181 = property on="initialize" class="Bool"("Désactivé"=u8 0) -> ()  [unwired: 2 in, 2 out]
      n182 = property on="Acquire" class="Bool"("Visible"=FALSE) -> ()  [unwired: 2 in, 2 out]
      n183 = property on="Setup" class="Bool"("Visible"=FALSE) -> ()  [unwired: 2 in, 2 out]
      n184 = local write "indicator"("" ("indicator")) -> ()
      n185 = local write "initialized ?"(FALSE ("initialized ?")) -> ()
      n186 = local write "Continuous"(FALSE ("Continuous")) -> ()
      n187 = local write "Close"(FALSE ("Close")) -> ()
      n188 = property on="Device Name" class="Ring (严格)"("Désactivé"=u8 0) -> ()  [unwired: 2 in, 2 out]
      n189 = property on="Continuous" class="Bool (严格)"("Visible"=FALSE) -> ()  [unwired: 2 in, 2 out]
      n190 = local write "Commande tab"(T1."Settings" ("Commande tab")) -> ()
    }
    frame #1 {
      # "Read Uniq ID"
      n191 = stacked-sequence {
        frame #0 {
          n192 = call "read detector uniq-id.vi"() -> ("nbr of components"=w369:i32, "UniqueID"=w368:string[], "Name"=w367:string[])  [unwired: 4 out]
          n193 = for {
            N: w369 -> [_]
            tunnel: w368 -> [w371]
            tunnel: w367 -> [w370]
            n194 = property on="Device Name" class="Ring (严格)"("Chaînes []"=w370) -> ()  [unwired: 2 in, 2 out]
            n195 = property on="Uniques ID" class="Ring (严格)"("Chaînes []"=w371) -> ()  [unwired: 2 in, 2 out]
          }
        }
      }
    }
    frame #2 {
      n196 = while {
        stop <- "initialize" stop-if-true
        n197 = local read "Device Name"() -> (w374:u16)
        n198 = local write "Uniques ID"(w374) -> ()
        n199 = local read "Close"() -> (w372:bool)
        n200 = Stop(stop? (T)=w372) -> ()
        n201 = Wait Until Next ms Multiple(millisecond multiple=u32 100 ("n millisecondes")) -> ()  [unwired: 1 out]
      }
    }
    frame #3 {
      n202 = stacked-sequence {
        tunnel: [_ w384 _ _] -> w377
        tunnel: [_ w383 _ _] -> w376
        frame #0 {
          n203 = local write "indicator"("Initializing ..." ("indicator")) -> ()
        }
        frame #1 {
          n204 = local read "Uniques ID"() -> (w381:u16)
          n205 = property on="Uniques ID" class="Ring (严格)"() -> ("Chaînes []"=w382:string[])  [unwired: 2 in, 2 out]
          n206 = Index Array(array=w382, index=w381) -> (element=w380:string)
          n207 = call "Initialize CCD.vi"("Unique id:"=w380) -> ("activeYPixels"=→"Y Pixels:":i32, "JYCCDLib.IJYCCDReqd"=w383:refnum<k7>, "activeXPixels"=→"X Pixels:":i32, "sortie d'erreur"=w384:errorcluster, "FirmwareVersion"=→"Firmware\nVersion":string)  [unwired: 3 out]
        }
        frame #2 {
          n208 = property on="initialize" class="Bool"("Désactivé"=u8 2) -> ()  [unwired: 2 in, 2 out]
          n209 = property on="Device Name" class="Ring (严格)"("Désactivé"=u8 2) -> ()  [unwired: 2 in, 2 out]
          n210 = local write "Continuous"(FALSE ("Continuous")) -> ()
          n211 = property on="Setup" class="Bool"("Visible"=TRUE) -> ()  [unwired: 2 in, 2 out]
        }
        frame #3 {
          n212 = local write "initialized ?"(TRUE ("initialized ?")) -> ()
          n213 = local write "indicator"("Initialized !" ("indicator")) -> ()
        }
      }
    }
    frame #4 {
      # "Actually not working"
      # "Read ADC and GAIN"
      n214 = case shown="真" "Constante de condition\n(Voir l'aide contextuelle)" {
        tunnel: w396 -> [_ w406]
        tunnel: w395 -> [_ w405]
        frame False {
        }
        frame True {
          # "Read Input supported trigger"
          n215 = call "Trigger - Get Supported Input.vi"("JYCCDLib.IJYCCDReqd"=w406, "Error Input"=w405) -> ("trigAddress"=w400:i32, "eventPtr"=w401:i32, "trigEventString"=w404:string, "trigSigType"=w403:i32, "trigSigTypeString"=w402:string)  [unwired: 4 out]
          n216 = local write "trigSigTypeString"(w402) -> ()
          n217 = local write "trigAddress"(w400) -> ()
          n218 = local write "Trigger Type :"(w401) -> ()
          n219 = local write "trigEventString"(w404) -> ()
          n220 = local write "Signal type :"(w403) -> ()
        }
      }
      n221 = call "Init ADC & Gain.vi"("JYCCDLib.IJYCCDReqd"=w396, "input error"=w395) -> ("ADC Number"=w394:i32[], "ADC description"=w399:string[], "Gain Number"=w397:i32[], "Gain description"=w398:string[])
      n222 = local write "Gain Number"(w397) -> ()
      n223 = local write "ADC Number"(w394) -> ()
      n224 = stacked-sequence {
        tunnel: w399 -> [w407 _]
        tunnel: w398 -> [_ w408]
        frame #0 {
          n225 = property on="ADC" class="Ring (严格)"("Chaînes []"=w407) -> ()  [unwired: 2 in, 2 out]
        }
        frame #1 {
          n226 = property on="GAIN" class="Ring (严格)"("Chaînes []"=w408) -> ()  [unwired: 2 in, 2 out]
        }
      }
    }
    frame #5 {
      # "IS multi Accumulation Supported ?"
      n227 = call "MultiAccu - Is Supported.vi"("Error In"=w415, "JYCCDLib.IJYCCDReqd"=w416) -> ("IsOperatingModeSupported"=w409:bool)  [unwired: 3 out]
      n228 = Select(t=0, s=w409, f=2) -> (s? t:f=w412:i32)
      n229 = Select(t=FALSE, s=w409, f=w409) -> (s? t:f=w411:bool)
      n230 = local write "Multi Accumulation mode:"(w411) -> ()
      n231 = property on="Multi Accumulation mode:" class="Bool (严格)"("Désactivé"=w412) -> ()  [unwired: 2 in, 2 out]
      n232 = property on="Multi Accumulation mode:" class="Bool (严格)"("Désactivé"=w412) -> ()  [unwired: 2 in, 2 out]
    }
    frame #6 {
      n233 = while {
        tunnel: w417 -> [w425]
        tunnel: w418 -> [w424]
        stop <- "Close" stop-if-true
        n234 = case shown="真" "Reformat" {
          frame False {
          }
          frame True {
            n235 = local read "Y Pixels:"() -> (w494:i32)
            n236 = local read "X Pixels:"() -> (w496:i32)
            n237 = call "Spectral Reformat CCD area.vi"("Y Pixels:"=w494, "X Pixels:"=w496, "numAreas"="Number of Areas :") -> ("areas :"=→"areas :":i32[][])  [unwired: 3 out]
          }
        }
        n238 = case shown="真" "Setup" {
          tunnel: w424 -> [_ w499]
          tunnel: w425 -> [_ w498]
          frame False {
          }
          frame True {
            n239 = stacked-sequence {
              tunnel: w499 -> [_ w513 _]
              tunnel: w498 -> [_ w501 _]
              frame #0 {
                n240 = local write "indicator"("Setting up the detector" ("indicator")) -> ()
              }
              frame #1 {
                w511 = 1 items=["JYMCD_ACQ_FORMAT_IMAGE", "JYMCD_ACQ_FORMAT_SCAN"] ("Acquisition type")
                n241 = local read "Gain Number"() -> (w506:i32[])
                n242 = local read "GAIN"() -> (w502:u16)
                n243 = local read "ADC Number"() -> (w507:i32[])
                n244 = local read "ADC"() -> (w503:u16)
                n245 = Index Array(array=w506, index=w502) -> (element=w504:i32)
                n246 = Index Array(array=w507, index=w503) -> (element=w505:i32)
                n247 = local read "Number of Areas :"() -> (w509:u16)
                n248 = local read "areas :"() -> (w510:i32[][])
                n249 = call "Setup CCD.vi"("numAreas"=w509, "areas :"=w510, "JYCCDLib.IJYCCDReqd"=w501, "entrée d'erreur (pas d'erreur)"=w513, "Acquisition type"=w511, "Gain"=w504, "Select ADC"=w505, "Integration time(ms)"="Integration time (ms) :") -> ("DataSize"=→"DataSize":i32)  [unwired: 1 out]
                "JYCCDLib.IJYCCDReqd" <- w501
              }
              frame #2 {
                w514 = TRUE ("Visible")
                n250 = property on="Continuous" class="Bool (严格)"("Visible"=w514) -> ()  [unwired: 2 in, 2 out]
                n251 = property on="Acquire" class="Bool"("Visible"=w514) -> ()  [unwired: 2 in, 2 out]
                n252 = local write "indicator"("Ready !" ("indicator")) -> ()
              }
            }
          }
        }
        n253 = local read "Continuous"() -> (w426:bool)
        n254 = local read "Accumulations:"() -> (w421:u16)
        n255 = Or(x="Acquire", y=w426) -> (x .or. y?=w423:bool)
        n256 = case shown="真" w423 {
          tunnel: w425 -> [_ w438]
          tunnel: w424 -> [_ w437]
          tunnel: "Enable InputTriggers :" -> [_ w436]
          tunnel: "Multi Accumulation mode:" -> [_ w435]
          tunnel: w421 -> [_ w434]
          tunnel: "MultiAcqShutterMode" -> [_ w433]
          frame False {
          }
          frame True {
            n257 = stacked-sequence {
              seq-local: [_ _ w451 _ _] -> [_ _ _ w479 _]
              tunnel: w438 -> [_ w440 w455 w478 _]
              tunnel: w437 -> [_ w441 w454 w477 _]
              tunnel: w436 -> [_ w442 _ _ _]
              tunnel: w435 -> [_ _ w453 _ _]
              tunnel: w434 -> [_ _ w452 _ _]
              tunnel: w433 -> [_ _ w450 _ _]
              frame #0 {
                n258 = local write "CCD Busy"(TRUE ("CCD Busy")) -> ()
              }
              frame #1 {
                n259 = case shown="真" w442 {
                  tunnel: w441 -> [w443 w449]
                  tunnel: w440 -> [w444 w448]
                  frame False {
                    n260 = call "Trigger - Disable.vi"("Error In"=w443, "JYCCDLib.IJYCCDReqd"=w444) -> ()  [unwired: 6 out]
                  }
                  frame True {
                    n261 = local read "Trigger Type :"() -> (w445:u16)
                    n262 = local read "Signal type :"() -> (w446:enum16{"TTL Rising Edge", "TTL Falling Edge"})
                    n263 = local read "trigAddress"() -> (w447:i32)
                    n264 = call "Trigger - Enable.vi"("Error In"=w449, "sigType"=w446, "event"=w445, "trigAddress"=w447, "JYCCDLib.IJYCCDReqd"=w448) -> ()  [unwired: 3 out]
                  }
                }
              }
              frame #2 {
                n265 = case shown="真" w453 {
                  selector: w453 -> [_ w461]
                  tunnel: w455 -> [w458 w464]
                  tunnel: w454 -> [w457 w463]
                  tunnel: w452 -> [_ w462]
                  tunnel: [u16 1 ("Accumulations:") w462] -> w451
                  tunnel: w450 -> [_ w460]
                  frame False {
                    n266 = call "MultiAccu - Disable.vi"("Error In"=w457, "JYCCDLib.IJYCCDReqd"=w458) -> ()  [unwired: 4 out]
                  }
                  frame True {
                    n267 = call "MultiAccu - Configure.vi"("JYCCDLib.IJYCCDReqd"=w464, "Cleans Before"="Number of Cleans", "Accumulations:"=w462, "MultiAcqHardwareMode"=w461, "MultiAcqShutterMode"=w460, "Error In"=w463) -> ()  [unwired: 1 in, 9 out]
                  }
                }
              }
              frame #3 {
                n268 = call "信号光谱2.vi"("error in"=w477, "Accumulations:"=w479, "ShutterOpen"="ShutterOpen", "JYCCDLib.IJYCCDReqd"=w478) -> ("Acq Time(ms)"=→"Acq Time(ms)":u32, "Array Out"=w476:i32[][][])  [unwired: 1 out]
                n269 = call "信号光谱2.vi"("Area Number"="Area Number to Display", "Array In"=w476) -> ("Array Out"=w474:i32[][])
                n270 = local read "Backlight"() -> (w473:i32[][])
                n271 = Subtract(x=w474, y=w473) -> (x-y=w471:i32[][])
                n272 = local write "Data"(w474) -> ()
                n273 = local write "data 2"(w471) -> ()
                n274 = Index Array(array=w471, index (row)=0 ("禁用的索引 (列)")) -> (element=w466:i32[])  [unwired: 1 in]
                n275 = local read "波长范围"() -> (w467:dbl[])
                n276 = Reverse 1D Array(array=w466) -> (reversed array=w465:i32[])
                n277 = call "转换至动态数据2"("Array"=w467) -> ("Dynamic Data Type"=w469:dynamicdata)  [unwired: 3 in]
                n278 = call "转换至动态数据"("Array"=w465) -> ("Dynamic Data Type"=w470:dynamicdata)  [unwired: 3 in]
                n279 = call "Build XY Graph2"("Y Input"=w470, "X Input"=w469) -> ("XY Graph"=w468:cluster{"Y":dbl[], "Y":dbl[]}[])  [unwired: 8 in, 1 out]
                n280 = local write "Spectrum"(w468) -> ()
              }
              frame #4 {
                n281 = case shown="真" "Save Backlight" {
                  frame False {
                  }
                  frame True {
                    n282 = local read "Data"() -> (w485:i32[][])
                    n283 = local write "Backlight"(w485) -> ()
                    n284 = local write "Save Backlight"(FALSE ("Save Backlight")) -> ()
                  }
                }
                n285 = local write "CCD Busy"(FALSE ("CCD Busy")) -> ()
              }
            }
          }
        }
        n286 = case shown="假" "Temperature" {
          tunnel: w425 -> [_ w488]
          tunnel: w424 -> [_ w487]
          frame False {
            n287 = property on="temp graph" class="WFChart (严格)"("Visible"=FALSE) -> ()  [unwired: 2 in, 2 out]
          }
          frame True {
            n288 = stacked-sequence {
              tunnel: w488 -> [_ w493]
              tunnel: w487 -> [_ w492]
              frame #0 {
                n289 = property on="temp graph" class="WFChart (严格)"("Visible"=TRUE) -> ()  [unwired: 2 in, 2 out]
              }
              frame #1 {
                w491 = u16 0 items=["° Celsius", "Kelvin", "° Farenheit"] ("units")
                n290 = call "read temperature.vi"("entrée d'erreur (pas d'erreur)"=w492, "units"=w491, "JYCCDLib.IJYCCDReqd"=w493) -> ("Current Temperature"=w490:dbl)
                n291 = local write "temp graph"(w490) -> ()
              }
            }
          }
        }
        n292 = Wait Until Next ms Multiple(millisecond multiple=u32 50 ("n millisecondes")) -> ()  [unwired: 1 out]
      }
    }
    frame #7 {
      n293 = Close Reference(reference=w517, error in (no error)=w516) -> ()  [unwired: 1 out]
    }
  }
  n294 = stacked-sequence {
    seq-local: [_ _ w527 _ _] -> [_ _ _ w537 w542]
    seq-local: [_ _ w526 _ _] -> [_ _ _ w536 _]
    seq-local: [_ _ _ w535 _] -> [_ _ _ _ _]
    frame #0 {
      n295 = call "信号光谱2.vi"() -> ("UniqueIDs"=w522:string[], "Mono ID"=w523:string[])  [unwired: 3 in, 1 out]
      n296 = Build Cluster Array(w523, w522) -> (w520:cluster{"String":string, "String":string}[])
      n297 = property on="Mono ID" class="CmbBox"("Strings And Values []"=w520) -> ()  [unwired: 2 in, 2 out]
      n298 = Index Array(array=w520, index=0) -> (element=w521:cluster{"String":string, "String":string})
      n299 = Unbundle(w521) -> ("String"=w518:string)  [unwired: 1 out]
      "Current UniqueID" <- w518
      n300 = local write "Mono ID"(w518) -> ()
    }
    frame #1 {
      n301 = while {
        stop <- "Connect" stop-if-true
        n302 = local read "Mono ID"() -> (w524:string)
        n303 = local write "Current UniqueID"(w524) -> ()
      }
    }
    frame #2 {
      n304 = local read "Mono ID"() -> (w529:string)
      n305 = call "信号光谱2.vi"("Unique ID"=w529, "Force Init"="Force\nInitialization") -> ("Refnum out"=w527:refnum<k7>, "Initialized"=→"Initialized JY":bool, "error out"=w526:errorcluster)  [unwired: 9 in, 2 out]
    }
    frame #3 {
      n306 = call "信号光谱2.vi"("Refnum in"=w537, "error in (no error)"=w536) -> ("Gratings"=w538:dbl[], "Grating Index"=w532:i32, "Current Grating"=w534:dbl, "Current Description"=w531:string, "error out"=w535:errorcluster)  [unwired: 5 in, 4 out]
      "Gratings" <- w538
      n307 = local write "Current Grating"(w534) -> ()
      n308 = local write "Current Description"(w531) -> ()
      n309 = Number To Decimal String(number=w538) -> (decimal integer string=w540:string[])  [unwired: 1 in]
      n310 = Number To Decimal String(number=w532) -> (decimal integer string=w533:string)  [unwired: 1 in]
      n311 = property on="Target Grating" class="CmbBox"("Value"=w533) -> ()  [unwired: 2 in, 2 out]
      n312 = Build Cluster Array(w540, string[] ["1", "2", "3"]) -> (w541:cluster{"Numeric":string, string}[])
      n313 = property on="Target Grating" class="CmbBox"("Strings And Values []"=w541) -> ()  [unwired: 2 in, 2 out]
    }
    frame #4 {
      n314 = while {
        tunnel: w542 -> [w544]
        stop <- w543 stop-if-true
        n315 = stacked-sequence {
          seq-local: [w548 _ _ _ _] -> [_ w555 w566 _ w573]
          seq-local: [w547 _ _ _ _] -> [_ w554 w565 _ _]
          seq-local: [_ w553 _ _ _] -> [_ _ _ _ _]
          seq-local: [_ w552 _ _ _] -> [_ _ _ _ _]
          seq-local: [_ _ w558 _ _] -> [_ _ _ _ _]
          seq-local: [_ _ w557 _ _] -> [_ _ _ w568 _]
          tunnel: w544 -> [w546 _ _ w569 _]
          frame #0 {
            n316 = call "信号光谱2.vi"("Refnum in"=w546) -> ("Grating Index"=→"Grating Index":i32, "Current Grating"=→"Current Grating":dbl, "Current Description"=→"Current Description":string, "error out"=w547:errorcluster, "JYMONOLib.IJYMonoReqd"=w548:refnum<k7>)  [unwired: 6 in, 4 out]
          }
          frame #1 {
            n317 = call "信号光谱2.vi"("error in (no error)"=w554, "JYMONOLib.IJYMonoReqd"=w555) -> ("error out"=w552:errorcluster, "Units"=→"Units":string, "Current WL"=→"Current WL":dbl, "JYMONOLib.IJYMonoReqd 2"=w553:refnum<k7>)  [unwired: 6 in]
          }
          frame #2 {
            w563 = u16 1 items=["Entrance", "Exit"] ("Mirror Number")
            w564 = u16 0 items=["Entrance", "Exit"] ("Mirror Number")
            n318 = call "信号光谱2.vi"("error in (no error)"=w565, "Mirror"=w564, "Refnum In"=w566) -> ("error out"=w561:errorcluster, "Current Mirror Position"=→"Entrance Mirror\nPosition":i32, "Refnum Out"=w562:refnum<k7>)  [unwired: 1 in]
            n319 = call "信号光谱2.vi"("error in (no error)"=w561, "Mirror"=w563, "Refnum In"=w562) -> ("error out"=w557:errorcluster, "Current Mirror Position"=→"Exit Mirror\nPosition":i32, "Refnum Out"=w558:refnum<k7>)  [unwired: 1 in]
          }
          frame #3 {
            w571 = u16 0 items=["Front Entrance", "Side Entrance", "Front Exit", "Side Exit", "First Intermediate", "Second Intermediate"] ("Slit")
            n320 = call "信号光谱2.vi"("MonoRefNum IN"=w569, "Slit"=w571, "error in (no error)"=w568) -> ("Units"=→"Units 2":string, "Slit Width"=→"Front Entrance":dbl, "error out"=→"error out":errorcluster)  [unwired: 13 in, 1 out]
          }
          frame #4 {
            n321 = local read "Move To\nTarget Positions"() -> (w574:bool)
            n322 = case shown="真" w574 {
              tunnel: w573 -> [_ w575]
              frame False {
              }
              frame True {
                n323 = stacked-sequence {
                  seq-local: [w577 _ _ _] -> [_ w583 _ _]
                  seq-local: [_ w581 _ _] -> [_ _ w598 _]
                  seq-local: [_ _ w585 _] -> [_ _ _ w604]
                  seq-local: [_ _ _ w601] -> [_ _ _ _]
                  tunnel: w575 -> [w579 w582 w596 w605]
                  frame #0 {
                    n324 = property on="Target Grating" class="CmbBox"() -> ("Value"=w576:string)  [unwired: 2 in, 2 out]
                    n325 = local read "error out"() -> (w578:errorcluster)
                    n326 = Decimal String To Number(string=w576) -> (number=w580:i32)  [unwired: 2 in, 1 out]
                    n327 = call "信号光谱2.vi"("error in (no error)"=w578, "Grating Index"=w580, "JYMONOLib.IJYMonoReqd"=w579) -> ("error out"=w577:errorcluster)  [unwired: 2 out]
                  }
                  frame #1 {
                    # "Move Grating to Target Position"
                    n328 = call "信号光谱2.vi"("error in (no error)"=w583, "Target WL"="Target WL", "RefNum In"=w582) -> ("error out"=w581:errorcluster)  [unwired: 1 in, 2 out]
                  }
                  frame #2 {
                    w591 = u16 1 items=["Entrance", "Exit"] ("Mirror Number")
                    w590 = u16 0 items=["Entrance", "Exit"] ("Mirror Number")
                    w597 = u16 1 items=["Entrance", "Exit", "Front", "Side"] ("Mirror Number")
                    w600 = u16 0 items=["Entrance", "Exit", "Front", "Side"] ("Mirror Number")
                    # "Move Mirrors"
                    n329 = call "信号光谱2.vi"("error in (no error)"=w598, "Mirror Position"="Entrance Mirror", "Mirror Number"=w600, "RefNum In"=w596) -> ("error out"=w595:errorcluster)  [unwired: 6 in, 1 out]
                    n330 = call "信号光谱2.vi"("error in (no error)"=w595, "Mirror Position"="Exit Mirror", "Mirror Number"=w597, "RefNum In"=w596) -> ("error out"=w588:errorcluster, "MonoRefNum Out"=w589:refnum<k7>)  [unwired: 6 in]
                    n331 = call "信号光谱2.vi"("error in (no error)"=w588, "Mirror"=w590, "Refnum In"=w589) -> ("error out"=w593:errorcluster, "Current Mirror Position"=w587:i32, "Refnum Out"=w592:refnum<k7>)  [unwired: 1 in]
                    n332 = local write "Entrance Mirror\nPosition"(w587) -> ()
                    n333 = call "信号光谱2.vi"("error in (no error)"=w593, "Mirror"=w591, "Refnum In"=w592) -> ("error out"=w585:errorcluster, "Current Mirror Position"=w586:i32)  [unwired: 1 in, 1 out]
                    n334 = local write "Exit Mirror\nPosition"(w586) -> ()
                  }
                  frame #3 {
                    w603 = u16 0 items=["Front Entrance", "Side Entrance", "Front Exit", "Side Exit", "First Intermediate", "Second Intermediate"] ("Slit")
                    # "Set New Slit Positions"
                    n335 = call "信号光谱2.vi"("JYMONOLib.IJYMonoReqd"=w605, "Slit"=w603, "error in (no error)"=w604, "Slit Width"="Target\nFront Entrance") -> ("error out"=w601:errorcluster)  [unwired: 1 in, 1 out]
                  }
                }
              }
            }
          }
        }
        n336 = local read "Close"() -> (w543:bool)
      }
    }
  }
  "Backlight" <- i32[][] [] ("Backlight")
  "data 2" <- i32[][] [] ("data 2")
